vi "IIC Read Bytes.vi"(5 "TimeOutMs":i32, 6 "ReadLen":i32, 7 "pReadData":u8, 9 "SlaveAddr":i16, 10 "IICIndex":i32, 11 "DevHandle":i32) -> (2 "function return":i32, 3 "pReadData out":u8)   [LabVIEW 2010, in "usb2iic.lvlib"]
doc: "int WINAPI IIC_ReadBytes(int DevHandle,int IICIndex,short SlaveAddr,unsigned char *pReadData,int ReadLen,int TimeOutMs);"
uses:
  usb2iic.lvlib
  USB2XXX.dll
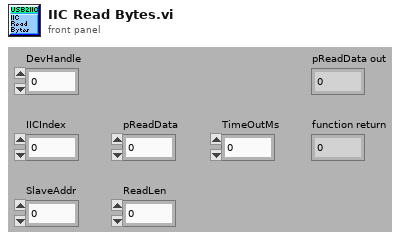
[diagram p1: front panel]
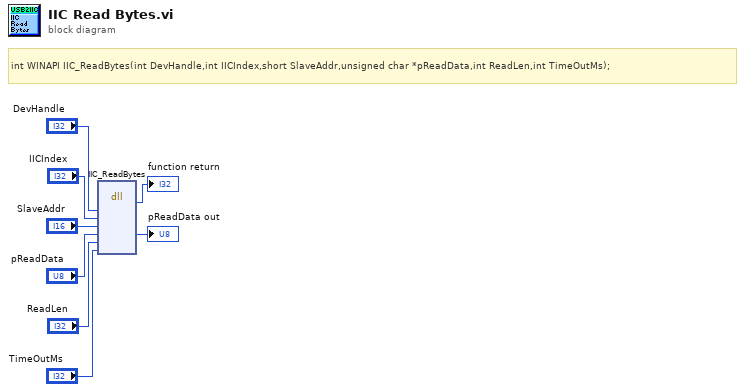
[diagram p0: block diagram]
diagram:
  # "int WINAPI IIC_ReadBytes(int DevHandle,int IICIndex,short SlaveAddr,unsigned char *pReadData,int ReadLen,int TimeOutMs);"
  n1 = dll-call lib="G:/OtherWork/USB2XXX_Example/trunk/Labview/PublicFiles/usb2iic/USB2XXX.*" fn="IIC_ReadBytes"("DevHandle"="DevHandle", "IICIndex"="IICIndex", "SlaveAddr"="SlaveAddr", "pReadData"="pReadData", "ReadLen"="ReadLen", "TimeOutMs"="TimeOutMs") -> (→"function return":i32, "pReadData"=→"pReadData out":u8)  [unwired: 8 in, 2 out]
